vi "FTW-Inbox-Destroy.vi"(0 "FTW Router":refnum<data-value>, 11 "error in":errorcluster) -> (15 "error out":errorcluster)   [LabVIEW 2014]
uses:
  core/FTW-Inbox-Core-Type.ctl
  json/core/FTW-JSON-Core-Structure.ctl
  core/FTW-Inbox-Core-IncomingMessageHeader.ctl
  error/FTW-ERR-ThrowGenericError.vi
  error/FTW-ERR-ThrowError.vi
  error/FTW-ERR-CallChain.vi
  string/FTW-STR-ReplaceWhitespace.vi
panel:
  # "Inputs"
  # "Outputs"
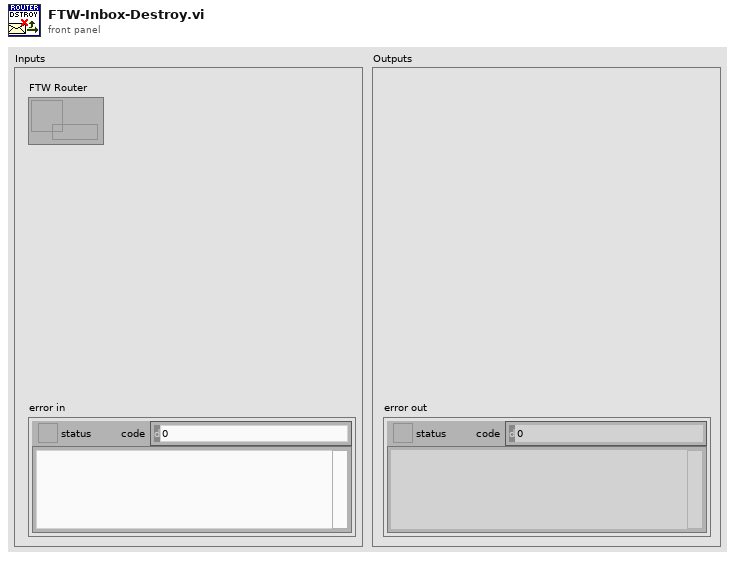
[diagram p1: front panel]
types:
  T1 = typedef "FTW-Inbox-Core-Type.ctl" = cluster{"Socket":i64, "MessageNotifier":refnum<user-event>, "Priority Brokers":refnum<user-event>[]}
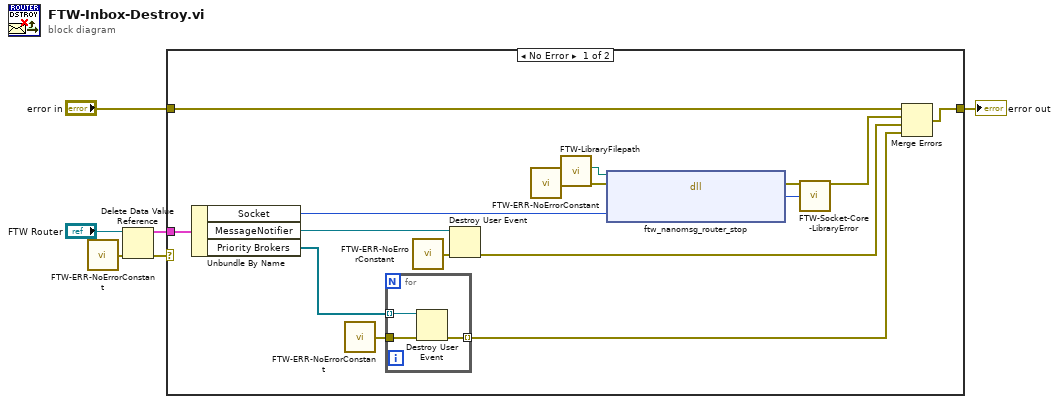
[diagram p0: block diagram]
diagram:
  n1 = call "FTW-ERR-NoErrorConstant.vi"() -> ("no error"=w1:errorcluster)
  n2 = Delete Data Value Reference(data value reference="FTW Router", error in=w1) -> (data value=w3:T1, error out=w2:errorcluster)
  n3 = case shown="No Error" w2 {
    tunnel: [w22 w26] -> w6
    tunnel: "error in" -> [w20 w26]
    tunnel: w3 -> [w14 _]
    frame No Error {
      n4 = Unbundle By Name(w14) -> ("Socket"=w19:i64, "MessageNotifier"=w18:refnum<user-event>, "Priority Brokers"=w17:refnum<user-event>[])
      n5 = call "FTW-ERR-NoErrorConstant.vi"() -> ("no error"=w15:errorcluster)
      n6 = for {
        tunnel: w17 -> [w25] mode=indexing
        tunnel: [w24] -> w12 mode=indexing
        tunnel: w15 -> [w23]
        n7 = Destroy User Event(user event=w25, error in=w23) -> (error out=w24:errorcluster)
      }
      n8 = call "FTW-ERR-NoErrorConstant.vi"() -> ("no error"=w16:errorcluster)
      n9 = Destroy User Event(user event=w18, error in=w16) -> (error out=w13:errorcluster)
      n10 = call "FTW-ERR-NoErrorConstant.vi"() -> ("no error"=w7:errorcluster)
      n11 = call "FTW-LibraryFilepath.vi"("error in"=w7) -> ("error out"=w8:errorcluster, "Library Filepath"=w11:path)  [unwired: 8 in, 1 out]
      n12 = dll-call lib="C:/Users/Jack/repo/ftw-master/Actor/src/Endpoint/Core/FTWLib-nanomsg32.dll" fn="ftw_nanomsg_router_stop"(path in=w11, error in=w8, "Socket Handle"=w19) -> (error out=w10:errorcluster, "Return Value"=w9:i64)  [unwired: 2 in, 1 out]
      n13 = call "FTW-Socket-Core-LibraryError.vi"("error in"=w10, "Return Value"=w9) -> ("error out"=w21:errorcluster)  [unwired: 13 in]
      n14 = Merge Errors(w20, w21, w13, w12) -> (w22:errorcluster)
    }
    frame Error {
    }
  }
  "error out" <- w6
